vi "Acquisition.vi"(8 "error in (no error)":errorcluster caption="entrée d'erreur (pas d'erreur)", 11 "Spectro Acq en entrée":refnum<class "Spectro Acquisition.lvclass">) -> (0 "error out":errorcluster caption="sortie d'erreur", 3 "Spectro Acq en sortie":refnum<class "Spectro Acquisition.lvclass">)   [LabVIEW 2024, in "Spectro Acquisition.lvclass"]
uses:
  Spectro Acquisition.lvclass
  Spectro Acquisition.lvclass/Spectro Acquisition.ctl
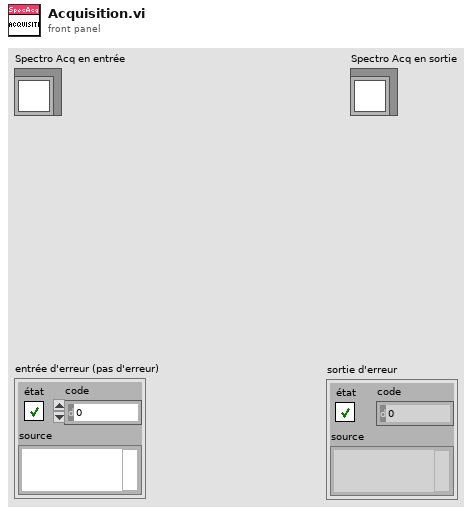
[diagram p1: front panel]
types:
  T1 = cluster{"Wavelenghts":dbl[], "Spectre-BKG":dbl[]}
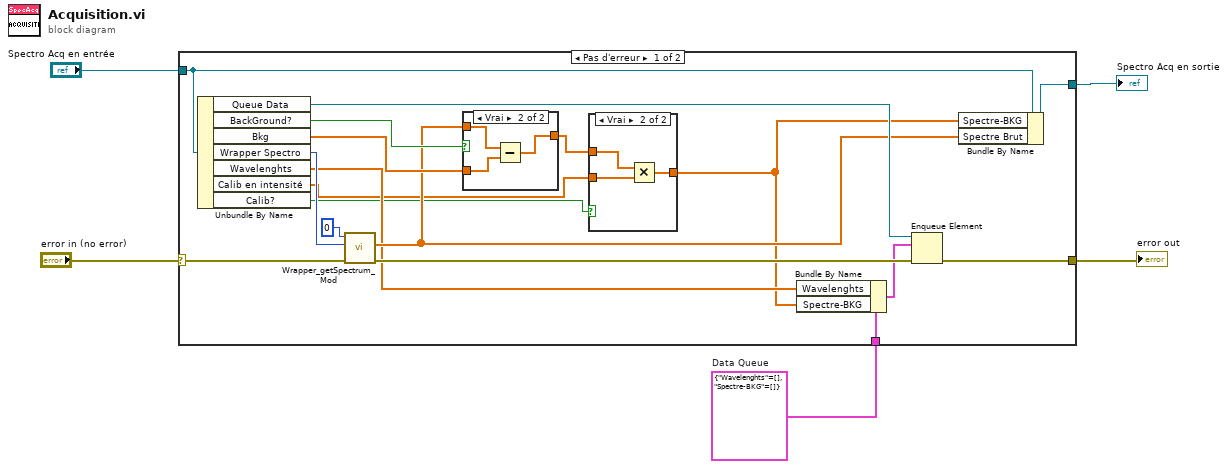
[diagram p0: block diagram]
diagram:
  w1 = T1 {"Wavelenghts"=[], "Spectre-BKG"=[]}  # Data Queue
  n1 = case shown="Pas d'erreur" "error in (no error)" {
    selector: "error in (no error)" -> [w22 w33]
    tunnel: [w15 w33] -> w4
    tunnel: [w13 w32] -> w2
    tunnel: "Spectro Acq en entrée" -> [w21 w32]
    tunnel: w1 -> [w10 _]
    frame No Error {
      n2 = Unbundle By Name(w21) -> ("Queue Data"=w17:refnum<queue>, "BackGround?"=w20:bool, "Bkg"=w19:dbl[], "Wrapper Spectro"=w18:u32, "Wavelenghts"=w11:dbl[], "Calib en intensité"=w6:dbl[], "Calib?"=w7:bool)
      n3 = call "Wrapper_getSpectrum_Mod.vi"("error in (no error)"=w22, "Wrapper"=w18, "Index"=0) -> ("error out"=w16:errorcluster, "Spectrum Values"=w12:dbl[])  [unwired: 6 in, 1 out]
      n4 = case shown="Vrai" w20 {
        tunnel: w19 -> [_ w31]
        tunnel: w12 -> [w28 w30]
        tunnel: [w28 w29] -> w9
        frame False {
        }
        frame True {
          n5 = Subtract(x=w30, y=w31) -> (x-y=w29:dbl[])
        }
      }
      n6 = case shown="Vrai" w7 {
        tunnel: w9 -> [w24 w27]
        tunnel: [w24 w26] -> w8
        tunnel: w6 -> [_ w25]
        frame False {
        }
        frame True {
          n7 = Multiply(x=w27, y=w25) -> (x*y=w26:dbl[])
        }
      }
      n8 = Bundle By Name(cluster=w10, "Wavelenghts"=w11, "Spectre-BKG"=w8) -> (w14:T1)
      n9 = Enqueue Element(queue=w17, element=w14, error in (no error)=w16) -> (error out=w15:errorcluster)  [unwired: 1 in, 2 out]
      n10 = Bundle By Name(cluster=w21, "Spectre-BKG"=w8, "Spectre Brut"=w12) -> (w13:refnum<class "Spectro Acquisition.lvclass">)
    }
    frame Error {
    }
  }
  "error out" <- w4
  "Spectro Acq en sortie" <- w2
